vi "DialogUsingEvents 2.vi"() -> (3 "Cancelled?":bool)   [LabVIEW 2018]
doc: "Use this template to create a dialog box with event handling."
panel:
  in  "Cancel":bool
  in  "OK":bool
  # "Add the contents of your dialog here.\n\nTip: use controls from the System category of the Controls \npalette for professional appearance.\n\nReplace this text with your own, or delete this label."
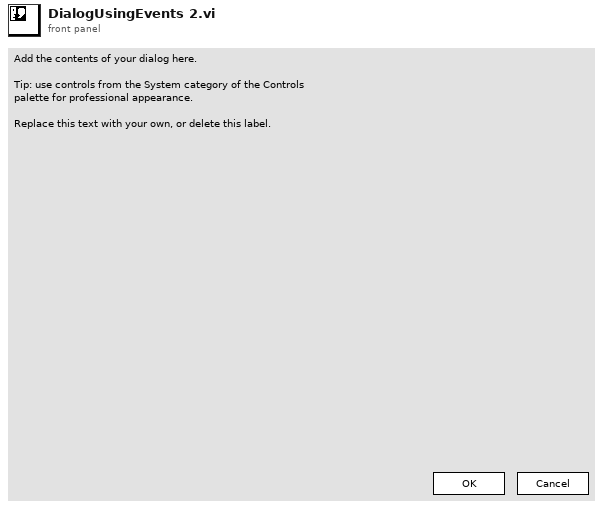
[diagram p1: front panel]
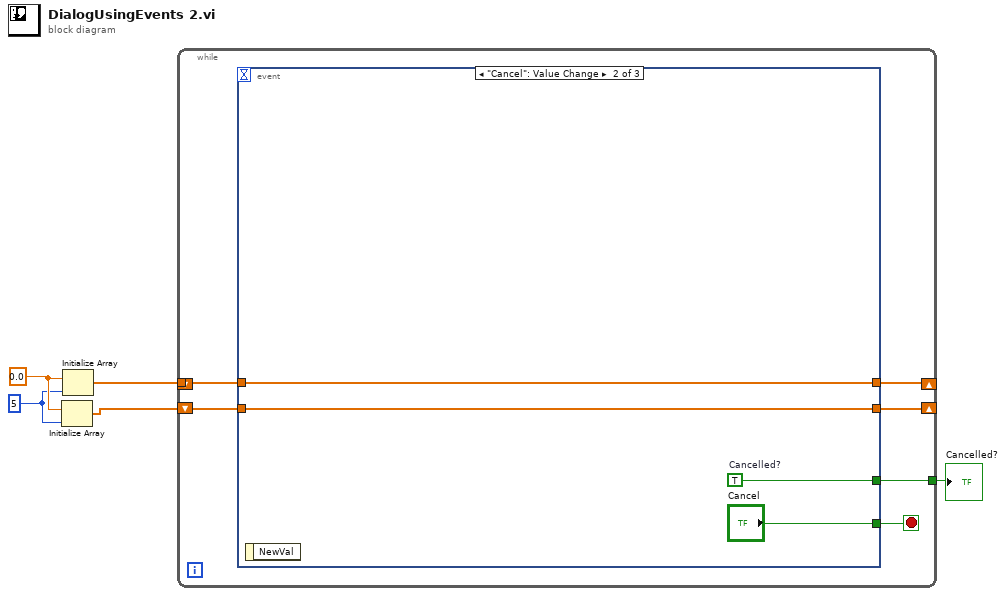
[diagram p0: block diagram]
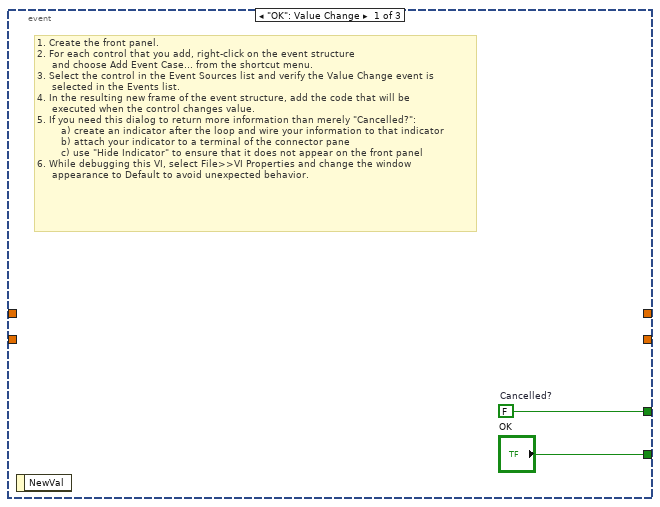
[diagram p2: hidden frame]
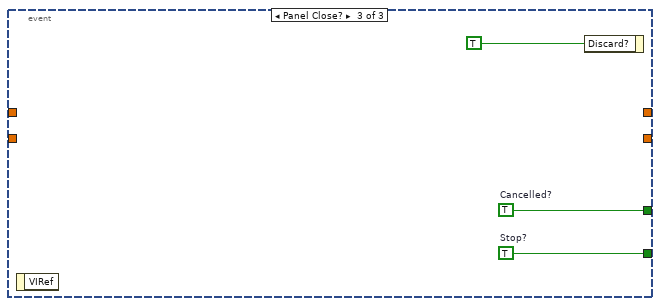
[diagram p3: hidden frame]
diagram:
  w3 = 5 ("dimension size")
  w4 = 0.0 ("element")
  n1 = Initialize Array(w4, w3) -> (w1:dbl[])
  n2 = Initialize Array(w4, w3) -> (w2:dbl[])
  n3 = while {
    tunnel: [w10] -> w5
    tunnel: w2 -> [w9]
    shift-right: [w6] -> _
    shift-left: w1 -> [w8]
    shift-right: [w7] -> _
    shift-left: _ -> [_]
    stop <- w11 stop-if-true
    n4 = event shown="[1] \"Cancel\": Value Change" {
      selector: _ -> [_ _ _]
      dyn-events: _ -> [_ _ _]
      timeout: _ -> [_ _ _]
      tunnel: ["OK" "Cancel" w19] -> w11
      tunnel: [w13 w17 w18] -> w10
      tunnel: w9 -> [_ w15 _]
      tunnel: w8 -> [_ w14 _]
      tunnel: [_ w15 _] -> w7
      tunnel: [_ w14 _] -> w6
      event "OK": Value Change {
        w13 = FALSE  # Cancelled?
        # "1. Create the front panel.\n2. For each control that you add, right-click on the event structure \n     and choose Add Event Case... from the shortcut menu.\n3. Select the control in the Event Sources list and verify the Value Change event is \n     selected in the Events list.\n4. In the resulting new frame of the event structure, add the code that will be \n     executed when the control changes value.\n5. If you need this dialog to return more information than merely \"Cancelled?\":\n        a) create an indicator after the loop and wire your information to that indicator\n        b) attach your indicator to a terminal of the connector pane\n        c) use \"Hide Indicator\" to ensure that it does not appear on the front panel\n6. While debugging this VI, select File>>VI Properties and change the window \n     appearance to Default to avoid unexpected behavior."
        n5 = event-data() -> ()  [unwired: 1 in, 1 out]
      }
      event "Cancel": Value Change {
        w17 = TRUE  # Cancelled?
        n6 = event-data() -> ()  [unwired: 1 in, 1 out]
      }
      event Panel Close? {
        w18 = TRUE  # Cancelled?
        w19 = TRUE  # Stop?
        n7 = event-data() -> ()  [unwired: 1 in, 1 out]
        n8 = event-data("Discard?"=TRUE) -> ()  [unwired: 1 in, 1 out]
      }
    }
  }
  "Cancelled?" <- w5
